vi "Shutdown.vi"(8 "error in (no error)":errorcluster, 11 "Oscilloscope in":refnum<class "Oscilloscope.lvclass">) -> (0 "error out":errorcluster, 3 "Oscilloscope out":refnum<class "Oscilloscope.lvclass">)   [LabVIEW 2018, in "Oscilloscope.lvlib" / "Oscilloscope.lvclass"]
doc: "This method shuts down the communication with the Oscope instrument by invoking the Disconnect.vi override."
uses:
  Oscilloscope.lvclass
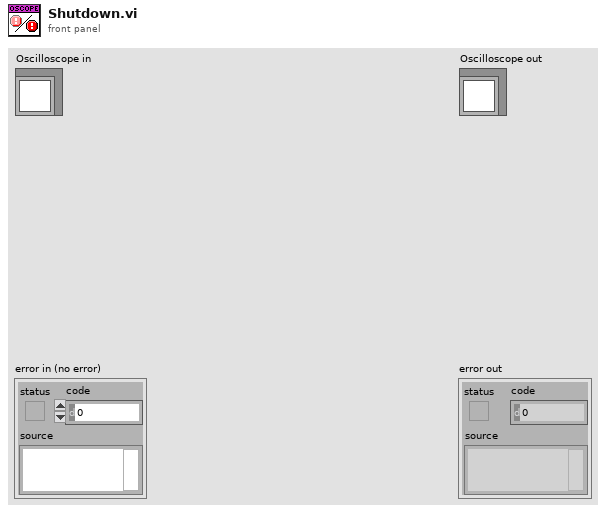
[diagram p1: front panel]
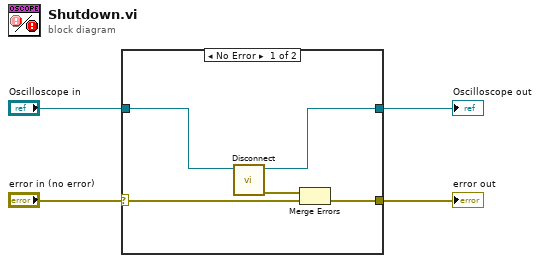
[diagram p0: block diagram]
diagram:
  n1 = case shown="No Error" "error in (no error)" {
    selector: "error in (no error)" -> [w7 w11]
    tunnel: [w5 w11] -> w3
    tunnel: [w8 w10] -> w1
    tunnel: "Oscilloscope in" -> [w9 w10]
    frame No Error {
      n2 = call-dynamic "Disconnect.vi"("Oscilloscope in"=w9) -> ("error out"=w6:errorcluster, "Oscilloscope out"=w8:refnum<class "Oscilloscope.lvclass">)  [unwired: 9 in]
      n3 = Merge Errors(w6, w7) -> (w5:errorcluster)
    }
    frame Error {
    }
  }
  "error out" <- w3
  "Oscilloscope out" <- w1
